vi "Page_Registry_Read.vi"(6 "ctlReferences":T1, 8 "error in (no error)":errorcluster, 11 "Class in":refnum<class "Installer.lvclass">) -> (0 "error out":errorcluster)   [LabVIEW 2020, in "Installer.lvclass"]
uses:
  <vilib>/AppBuilder/IB_Classes/Installer/Installer.lvclass
  <resource>/Framework/Providers/Builds/Installer/Pages/controls/IB_UI_Page_Registry_References.ctl
  <resource>/Framework/Providers/Builds/Installer/CDK_sTypeDef_NewFolder.ctl
  <resource>/Framework/Providers/Builds/Installer/CDK_sTypeDef_Remove.ctl
  <resource>/Framework/Providers/Builds/Installer/CDK_sTypeDef_Add.ctl
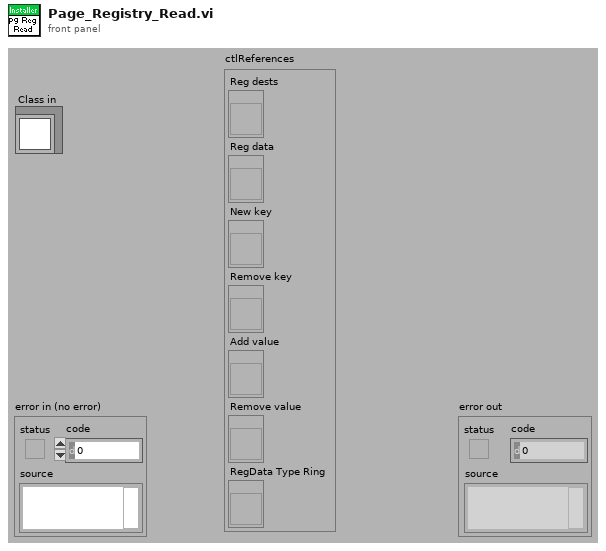
[diagram p1: front panel]
types:
  T1 = typedef "IB_UI_Page_Registry_References.ctl" = cluster{"Reg dests":refnum<vi>, "Reg data":refnum<vi>, "New key":refnum<vi>, "Remove key":refnum<vi>, "Add value":refnum<vi>, "Remove value":refnum<vi>, "RegData Type Ring":refnum<vi>}
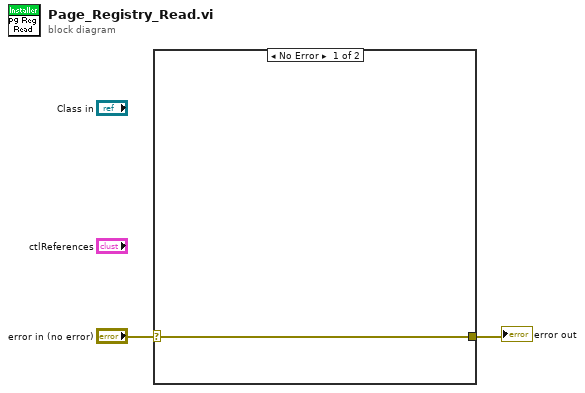
[diagram p0: block diagram]
diagram:
  n1 = case shown="No Error" "error in (no error)" {
    selector: "error in (no error)" -> [w3 w4]
    tunnel: [w3 w4] -> w1
    frame No Error {
    }
    frame Error {
    }
  }
  "error out" <- w1
